vi "NewtonsPSM_Speed&Smoothing.vi"(0 "VISA session":refnum<visa-resource-name>, 1 "Windows Size (0,01)":sgl=0.01 min=0.01 max=10 step=0.01 format="%#_6f", 2 "Minimum Cycles (1)":u16=1 min=1 step=1, 3 "Delay (0)":u16 max=60 step=1, 5 "Acquisition Speed (Medium)":u16(ring)=1 items=["FAST", "MEDIUM", "SLOW", "VERY SLOW", "WINDOW"], 7 "Smothing filter (Normal)":u16(ring)=1 items=["NONE", "NORMAL", "SLOW"], 9 "Smothing response (Auto)":u16(ring) items=["AUTO", "FIXED"], 11 "error in (no error)":errorcluster, 12 "Phase Reference (CH1)":u16(ring) items=["CH1", "CH2"], 13 "Low Frequency (Off)":bool) -> (4 "dup VISA session":refnum<visa-resource-name>, 15 "error out":errorcluster)   [LabVIEW 2025, in "NewtonsPSM1735.lvlib"]
doc: "This VI set the configuration for the acquisiation parameter of the PSM 1735.\nAcquisition Speed, Smoothing filter parameters, and reference parameters."
uses:
  NewtonsPSM1735.lvlib
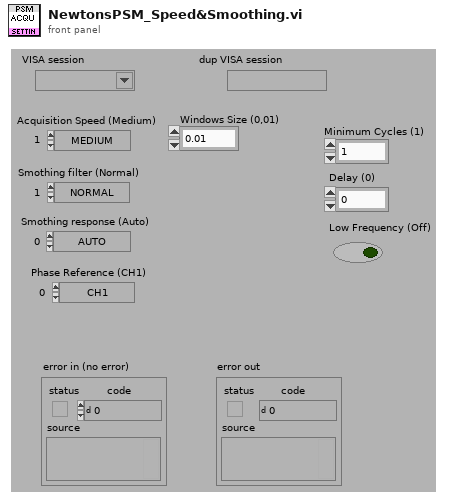
[diagram p1: front panel]
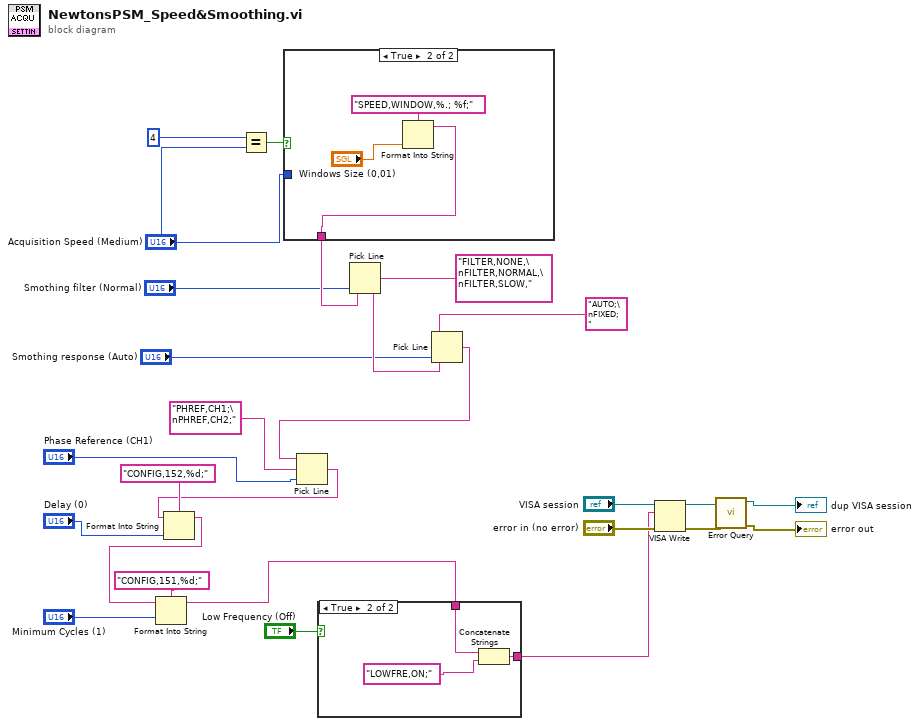
[diagram p0: block diagram]
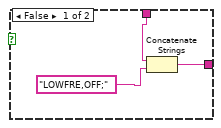
[diagram p2: hidden frame]
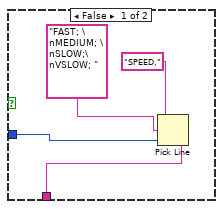
[diagram p3: hidden frame]
diagram:
  n1 = Equal?(x=4, y="Acquisition Speed (Medium)") -> (x = y?=w20:bool)
  n2 = case shown="True" w20 {
    tunnel: [w30 w32] -> w25
    tunnel: "Acquisition Speed (Medium)" -> [w28 _]
    frame False {
      n3 = Pick Line(string ("")="SPEED,", multi-line string="FAST; \nMEDIUM; \nSLOW;\nVSLOW; ", line index=w28) -> (output string=w30:string)
    }
    frame True {
      n4 = Format Into String(format string="SPEED,WINDOW,%.; %f;", "Windows Size (0,01)") -> (resulting string=w32:string)  [unwired: 2 in, 1 out]
    }
  }
  n5 = Pick Line(string ("")=w25, multi-line string="FILTER,NONE,\nFILTER,NORMAL,\nFILTER,SLOW,", line index="Smothing filter (Normal)") -> (output string=w23:string)
  n6 = Pick Line(string ("")=w23, multi-line string="AUTO;\nFIXED; ", line index="Smothing response (Auto)") -> (output string=w9:string)
  n7 = Pick Line(string ("")=w9, multi-line string="PHREF,CH1;\nPHREF,CH2;" ("chaîne multiligne"), line index="Phase Reference (CH1)") -> (output string=w5:string)
  n8 = Format Into String(format string="CONFIG,152,%d;", initial string=w5, "Delay (0)") -> (resulting string=w3:string)  [unwired: 1 in, 1 out]
  n9 = Format Into String(format string="CONFIG,151,%d;", initial string=w3, "Minimum Cycles (1)") -> (resulting string=w1:string)  [unwired: 1 in, 1 out]
  n10 = case shown="True" "Low Frequency (Off)" {
    tunnel: [w36 w39] -> w15
    tunnel: w1 -> [w35 w38]
    frame False {
      n11 = Concatenate Strings(w35, "LOWFRE,OFF;") -> (w36:string)
    }
    frame True {
      n12 = Concatenate Strings(w38, "LOWFRE,ON;") -> (w39:string)
    }
  }
  n13 = VISA Write(VISA resource name="VISA session", write buffer=w15, error in (no error)="error in (no error)") -> (VISA resource name out=w13:refnum<visa-resource-name>, error out=w14:errorcluster)  [unwired: 1 out]
  n14 = call "Error Query.vi"("error in (no error)"=w14, "VISA resource name"=w13) -> ("error out"=→"error out":errorcluster, "VISA resource name out"=→"dup VISA session":refnum<visa-resource-name>)  [unwired: 8 out]
